vi "STOP.vi"(8 "error in (no error)":errorcluster caption="entrée d'erreur (pas d'erreur)", 11 "UV-VIS en entrée":refnum<class "CCD_camera.lvclass">) -> (0 "error out":errorcluster caption="sortie d'erreur", 3 "UV-VIS en sortie":refnum<class "CCD_camera.lvclass">)   [LabVIEW 2019, in "CCD_camera.lvclass"]
uses:
  CCD_camera.lvclass
  C:/Users/elysium/Documents/dev/TRANCON/Classes/GeneralFunctionality/GeneralFunctionality.lvclass
  GeneralFunctionality/GeneralFunctionality.lvclass/GeneralFunctionality.ctl
  GeneralFunctionality/GeneralFunctionality.lvclass
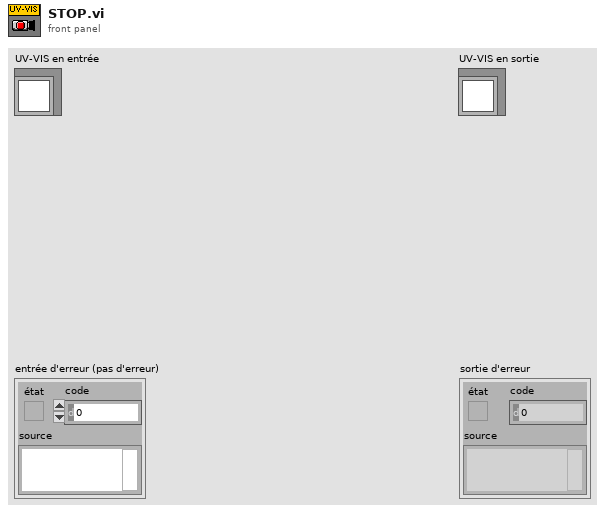
[diagram p1: front panel]
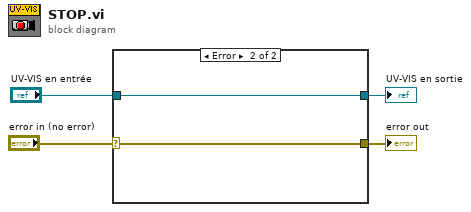
[diagram p0: block diagram]
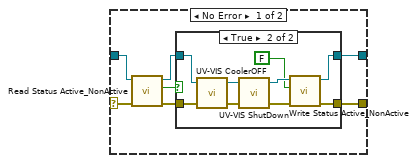
[diagram p2: hidden frame]
diagram:
  n1 = case shown="Error" "error in (no error)" {
    selector: "error in (no error)" -> [w5 w24]
    tunnel: "UV-VIS en entrée" -> [w8 w23]
    tunnel: [w7 w23] -> w3
    tunnel: [w6 w24] -> w2
    frame No Error {
      n2 = call "Read Status Active_NonActive.vi"("error in (no error)"=w5, "GeneralFunctionality in"=w8) -> ("error out"=w11:errorcluster, "Status Active/NonActive"=w9:bool, "GeneralFunctionality out"=w10:refnum<class "CCD_camera.lvclass">)  [unwired: 7 in]
      n3 = case shown="True" w9 {
        tunnel: [w12 w15] -> w6
        tunnel: [w13 w16] -> w7
        tunnel: w10 -> [w13 w18]
        tunnel: w11 -> [w12 w17]
        frame False {
        }
        frame True {
          n4 = call "UV-VIS CoolerOFF.vi"("error in (no error)"=w17, "UV-VIS  in"=w18) -> ("error out"=w19:errorcluster, "UV-VIS  out"=w20:refnum<class "CCD_camera.lvclass">)  [unwired: 1 in, 1 out]
          n5 = call "UV-VIS ShutDown.vi"("error in (no error)"=w19, "UV-VIS  in"=w20) -> ("error out"=w21:errorcluster, "UV-VIS  out"=w22:refnum<class "CCD_camera.lvclass">)  [unwired: 1 in, 1 out]
          n6 = call "Write Status Active_NonActive.vi"("error in (no error)"=w21, "Status Active/NonActive"=FALSE, "GeneralFunctionality in"=w22) -> ("error out"=w15:errorcluster, "GeneralFunctionality out"=w16:refnum<class "CCD_camera.lvclass">)  [unwired: 7 in]
        }
      }
    }
    frame Error {
    }
  }
  "error out" <- w2
  "UV-VIS en sortie" <- w3
